vi "set Command Data Element.vi"(8 "error in (no error)":errorcluster, 10 "Command Data Element":T1, 11 "REx - CMD_TEMPLATE in":refnum<class "Alpha Cmd.lvclass">) -> (0 "error out":errorcluster, 3 "REx - CMD_TEMPLATE out":refnum<class "Alpha Cmd.lvclass">)   [LabVIEW 2012, in "Alpha Cmd.lvclass"]
uses:
  Alpha Cmd.lvclass
  STYP - Command Data Element.ctl
  Alpha Cmd.lvclass/Alpha Cmd.ctl
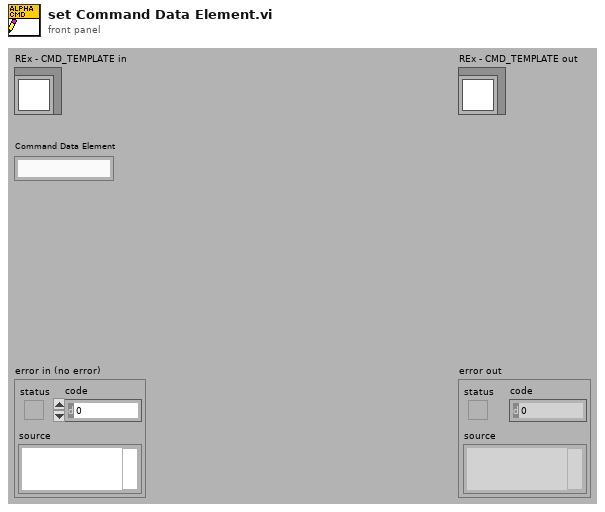
[diagram p1: front panel]
types:
  T1 = typedef "Alpha Cmd.lvclass/STYP - Command Data Element.ctl" = string
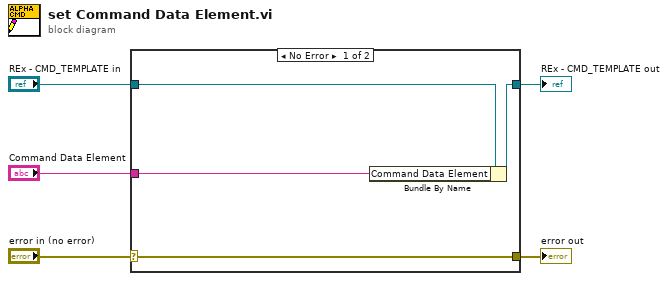
[diagram p0: block diagram]
diagram:
  n1 = case shown="No Error" "error in (no error)" {
    selector: "error in (no error)" -> [w9 w10]
    tunnel: [w9 w10] -> w4
    tunnel: [w7 w11] -> w2
    tunnel: "REx - CMD_TEMPLATE in" -> [w8 w11]
    tunnel: "Command Data Element" -> [w6 _]
    frame No Error {
      n2 = Bundle By Name(cluster=w8, "Command Data Element"=w6) -> (w7:refnum<class "Alpha Cmd.lvclass">)
    }
    frame Error {
    }
  }
  "error out" <- w4
  "REx - CMD_TEMPLATE out" <- w2
